vi "SwitchesMirrors Delays.vi"(2 "Set Switch":T1, 3 "Delays (ms)":cluster{"Laser":u32, "Video":u32}={"Laser"=500, "Video"=1500}, 4 "Status":T1) -> (0 "Delay":u32)   [LabVIEW 2014]
uses:
  SwitchesMirrors Status.ctl
panel:
  # "LICENSED MATERIALS – PROPERTY OF IBM\nCopyright IBM Corp. 2016,\nALL RIGHTS RESERVED"
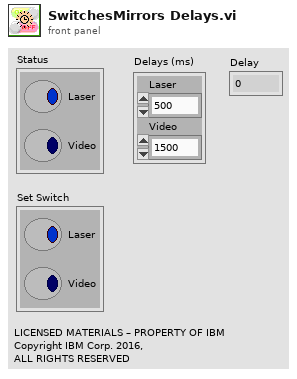
[diagram p1: front panel]
types:
  T1 = typedef "SwitchesMirrors Status.ctl" = cluster{"Laser":bool, "Video":bool}
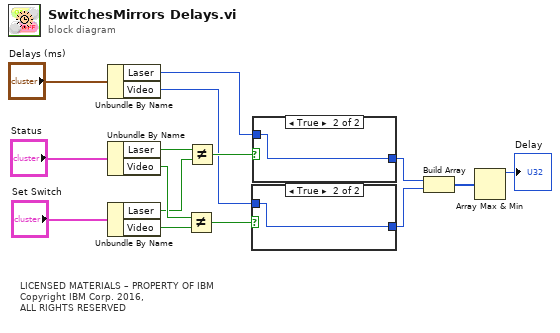
[diagram p0: block diagram]
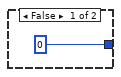
[diagram p2: hidden frame]
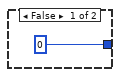
[diagram p3: hidden frame]
diagram:
  # "LICENSED MATERIALS – PROPERTY OF IBM\nCopyright IBM Corp. 2016,\nALL RIGHTS RESERVED"
  n1 = Unbundle By Name("Delays (ms)") -> ("Laser"=w4:u32, "Video"=w3:u32)
  n2 = Unbundle By Name("Status") -> ("Laser"=w9:bool, "Video"=w12:bool)
  n3 = Unbundle By Name("Set Switch") -> ("Laser"=w10:bool, "Video"=w13:bool)
  n4 = Not Equal?(x=w12, y=w13) -> (x != y?=w11:bool)
  n5 = Not Equal?(x=w9, y=w10) -> (x != y?=w8:bool)
  n6 = case shown="True" w11 {
    tunnel: [u32 0 ("milliseconds to wait") w17] -> w15
    tunnel: w3 -> [_ w17]
    frame False {
    }
    frame True {
    }
  }
  n7 = case shown="True" w8 {
    tunnel: [u32 0 ("milliseconds to wait") w19] -> w14
    tunnel: w4 -> [_ w19]
    frame False {
    }
    frame True {
    }
  }
  n8 = Build Array(w14, w15) -> (w2:u32[])
  n9 = Array Max & Min(array=w2) -> (max value=→"Delay":u32)  [unwired: 3 out]
